vi "BINHDR_H_write.vi"(8 "error in (no error)":errorcluster, 10 "BINHDR_H":T1, 11 "refnum in":refnum<file>) -> (0 "error out":errorcluster, 3 "refnum out":refnum<file>)   [LabVIEW 2012]
uses:
  TTTR_data_headers/BINHDR_H.ctl
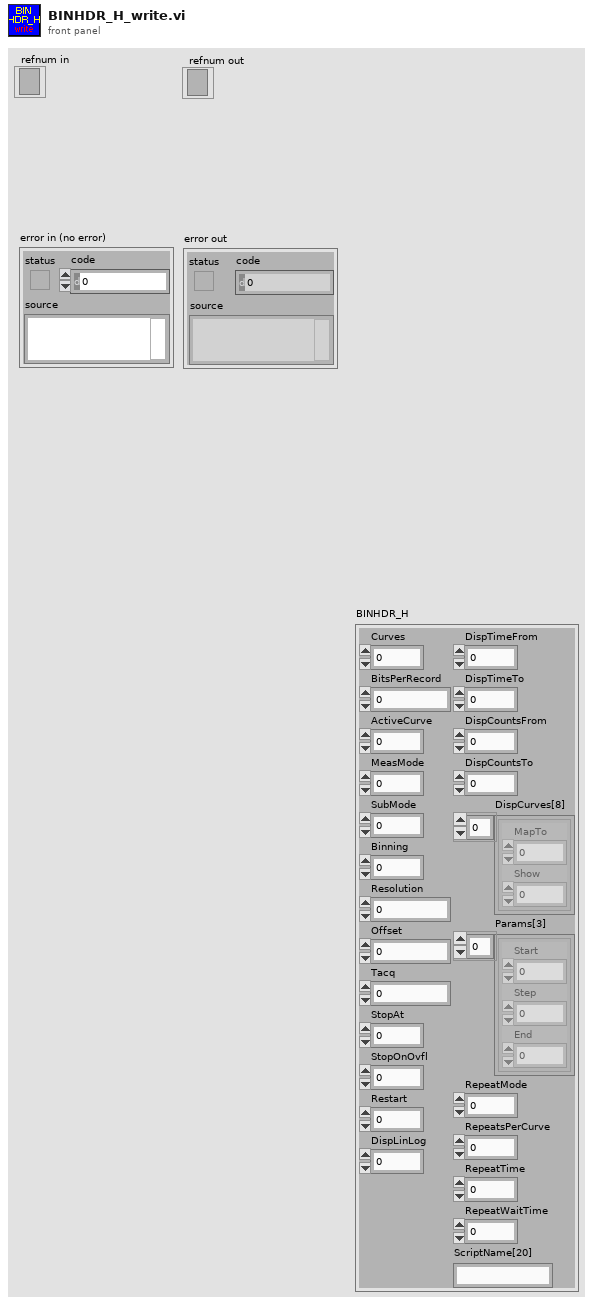
[diagram p1: front panel]
types:
  T1 = typedef "BINHDR_H.ctl" = cluster{"Curves":i32, "BitsPerRecord":i32, "ActiveCurve":i32, "MeasMode":i32, "SubMode":i32, "Binning":i32, "Resolution":dbl, "Offset":i32, "Tacq":i32, "StopAt":i32, "StopOnOvfl":i32, "Restart":i32, "DispLinLog":i32, "DispTimeFrom":i32, "DispTimeTo":i32, "DispCountsFrom":i32, "DispCountsTo":i32, "DispCurves[8]":cluster{"MapTo":i32, "Show":i32}[], "Params[3]":cluster{"Start":sgl, "Step":sgl, "End":sgl}[], "RepeatMode":i32, "RepeatsPerCurve":i32, "RepeatTime":i32, "RepeatWaitTime":i32, "ScriptName[20]":string}
  T2 = enum16{"big-endian, network order", "native, host order", "little-endian"}
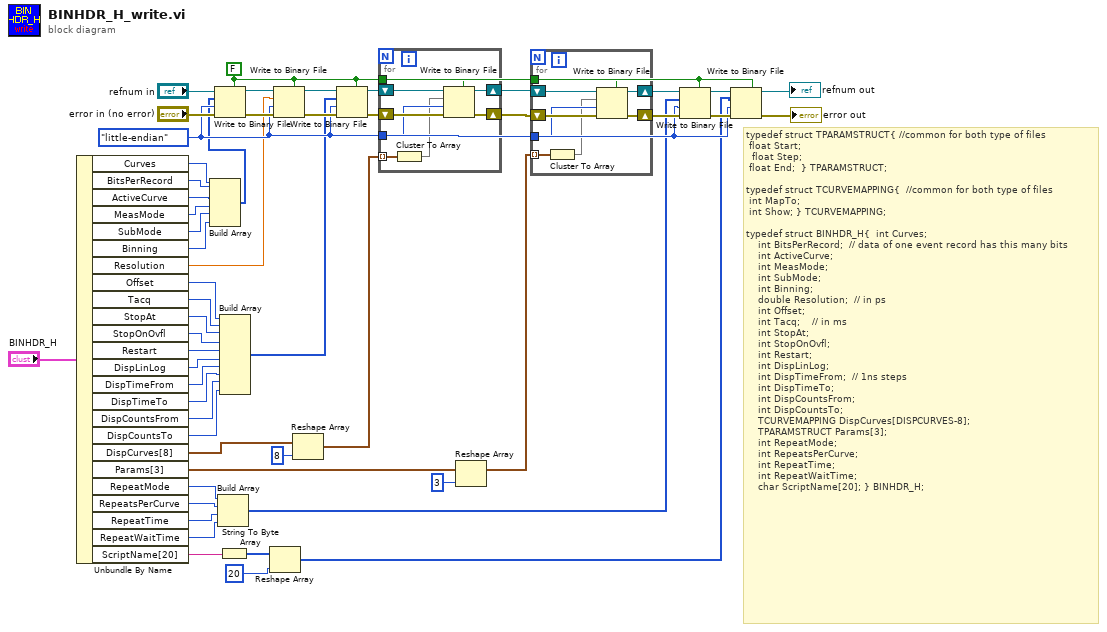
[diagram p0: block diagram]
diagram:
  w15 = FALSE ("prepend array or string size? (T)")
  w37 = T2."little-endian" ("byte order (0:big-endian, network order)")
  # "typedef struct TPARAMSTRUCT{\t//common for both type of files\n\tfloat Start;\n  float Step;\n\tfloat End;  } TPARAMSTRUCT;\n\ntypedef struct TCURVEMAPPING{\t\t//common for both type of files\n\tint MapTo;\n\tint Show; } TCURVEMAPPING;\n\ntypedef struct BINHDR_H{\t\tint Curves;\n\t\t\t\tint BitsPerRecord;\t\t// data of one event record has this many bits\n\t\t\t\tint ActiveCurve;\n\t\t\t\tint MeasMode;\n\t\t\t\tint SubMode;\n\t\t\t\tint Binning;\t\t\t\n\t\t\t\tdouble Resolution;\t\t// in ps\n\t\t\t\tint Offset;\t\t\t\t\n\t\t\t\tint Tacq;\t\t\t\t// in ms\n\t\t\t\tint StopAt;\n\t\t\t\tint StopOnOvfl;\n\t\t\t\tint Restart;\n\t\t\t\tint DispLinLog;\n\t\t\t\tint DispTimeFrom;\t\t// 1ns steps\n\t\t\t\tint DispTimeTo;\n\t\t\t\tint DispCountsFrom;\n\t\t\t\tint DispCountsTo;\n\t\t\t\tTCURVEMAPPING DispCurves[DISPCURVES-8];\t\n\t\t\t\tTPARAMSTRUCT Params[3];\n\t\t\t\tint RepeatMode;\n\t\t\t\tint RepeatsPerCurve;\n\t\t\t\tint RepeatTime;\n\t\t\t\tint RepeatWaitTime;\n\t\t\t\tchar ScriptName[20];\t} BINHDR_H;"
  n1 = Unbundle By Name("BINHDR_H") -> ("Curves"=w35:i32, "BitsPerRecord"=w34:i32, "ActiveCurve"=w33:i32, "MeasMode"=w32:i32, "SubMode"=w31:i32, "Binning"=w30:i32, "Resolution"=w28:dbl, "Offset"=w27:i32, "Tacq"=w26:i32, "StopAt"=w25:i32, "StopOnOvfl"=w24:i32, "Restart"=w23:i32, "DispLinLog"=w22:i32, "DispTimeFrom"=w21:i32, "DispTimeTo"=w20:i32, "DispCountsFrom"=w19:i32, "DispCountsTo"=w18:i32, "DispCurves[8]"=w16:cluster{"MapTo":i32, "Show":i32}[], "Params[3]"=w14:cluster{"Start":sgl, "Step":sgl, "End":sgl}[], "RepeatMode"=w13:i32, "RepeatsPerCurve"=w12:i32, "RepeatTime"=w11:i32, "RepeatWaitTime"=w10:i32, "ScriptName[20]"=w8:string)
  n2 = Build Array(w35, w34, w33, w32, w31, w30) -> (w29:i32[])
  n3 = Write to Binary File(file (use dialog)="refnum in", data=w29, error in="error in (no error)", 5:w15, 9:w37) -> (refnum out=w50:refnum<file>, error out=w51:errorcluster)  [unwired: 1 in, 1 out]
  n4 = Build Array(w13, w12, w11, w10) -> (w9:i32[])
  n5 = String To Byte Array(string=w8) -> (unsigned byte array=w7:u8[])
  n6 = Build Array(w27, w26, w25, w24, w23, w22, w21, w20, w19, w18) -> (w17:i32[])
  n7 = Reshape Array(w7, 20 ("count (1)")) -> (w5:u8[])
  n8 = Write to Binary File(file (use dialog)=w50, data=w28, error in=w51, 5:w15, 9:w37) -> (refnum out=w48:refnum<file>, error out=w49:errorcluster)  [unwired: 1 in, 1 out]
  n9 = Reshape Array(w16, 8) -> (w4:cluster{"MapTo":i32, "Show":i32}[])
  n10 = Write to Binary File(file (use dialog)=w48, data=w17, error in=w49, 5:w15, 9:w37) -> (refnum out=w46:refnum<file>, error out=w47:errorcluster)  [unwired: 1 in, 1 out]
  n11 = for {
    shift-right: [w58] -> w44
    shift-left: w47 -> [w61]
    shift-right: [w59] -> w45
    shift-left: w46 -> [w60]
    tunnel: w37 -> [w57]
    tunnel: w4 -> [w55] mode=indexing
    tunnel: w15 -> [w56]
    n12 = Cluster To Array(cluster=w55) -> (array=w54:i32[])
    n13 = Write to Binary File(file (use dialog)=w60, data=w54, error in=w61, 5:w56, 9:w57) -> (refnum out=w59:refnum<file>, error out=w58:errorcluster)  [unwired: 1 in, 1 out]
  }
  n14 = Reshape Array(w14, 3) -> (w2:cluster{"Start":sgl, "Step":sgl, "End":sgl}[])
  n15 = for {
    shift-right: [w67] -> w42
    shift-left: w44 -> [w69]
    shift-right: [w66] -> w43
    shift-left: w45 -> [w68]
    tunnel: w37 -> [w65]
    tunnel: w15 -> [w64]
    tunnel: w2 -> [w63] mode=indexing
    n16 = Cluster To Array(cluster=w63) -> (array=w62:sgl[])
    n17 = Write to Binary File(file (use dialog)=w68, data=w62, error in=w69, 5:w64, 9:w65) -> (refnum out=w66:refnum<file>, error out=w67:errorcluster)  [unwired: 1 in, 1 out]
  }
  n18 = Write to Binary File(file (use dialog)=w43, data=w9, error in=w42, 5:w15, 9:w37) -> (refnum out=w40:refnum<file>, error out=w41:errorcluster)  [unwired: 1 in, 1 out]
  n19 = Write to Binary File(file (use dialog)=w40, data=w5, error in=w41, 5:w15, 9:w37) -> (refnum out=→"refnum out":refnum<file>, error out=→"error out":errorcluster)  [unwired: 1 in, 1 out]
